vi "Write Numeric Scalar to Source (Base08 I8).vi"(8 "width (-)":i16, 9 "offset":i32, 10 "value":i8, 11 "error in":errorcluster) -> (1 "new offset":i32, 3 "error out":errorcluster)   [LabVIEW 2027, in "Static Errors.lvlib"]
doc: "Converts <b>value</b> into an octal-formatted string, and writes the string to the <b>error in</b> source buffer at the specified <b>offset</b>."
uses:
  Static Errors.lvlib
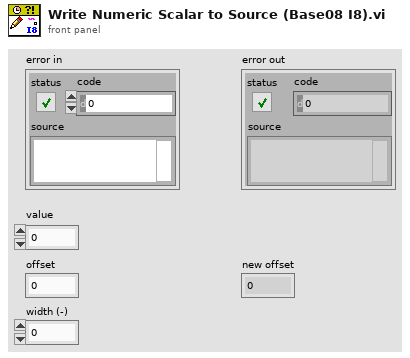
[diagram p1: front panel]
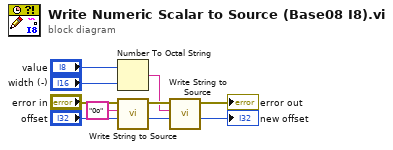
[diagram p0: block diagram]
diagram:
  n1 = Number To Octal String(1:"width (-)", 2:"value") -> (0:w2:string)
  n2 = call "Write String to Source.vi"("offset"="offset", "string"="0o", "error in"="error in") -> ("new offset"=w4:i32, "error out"=w3:errorcluster)  [unwired: 7 in]
  n3 = call "Write String to Source.vi"("offset"=w4, "string"=w2, "error in"=w3) -> ("new offset"=→"new offset":i32, "error out"=→"error out":errorcluster)  [unwired: 7 in]
